vi "getAdditionalDataFromXML.vi"(8 "error in (no error)":errorcluster, 10 "Xml":refnum<class "xmlNode.lvclass">, 11 "SingleToneRamp in":refnum<class "SingleToneRamp.lvclass">) -> (0 "error out":errorcluster, 2 "Xml out":refnum<class "xmlNode.lvclass">, 3 "SingleToneRamp out":refnum<class "SingleToneRamp.lvclass">)   [LabVIEW 2009, in "Tools.lvlib" / "Scripting.lvlib" / "SingleToneRamp.lvclass"]
uses:
  SingleToneRamp.lvclass
  xmlNode/xmlNode.lvclass
  SingleToneRamp.lvclass/SingleToneRamp.ctl
  SingleTone.lvclass
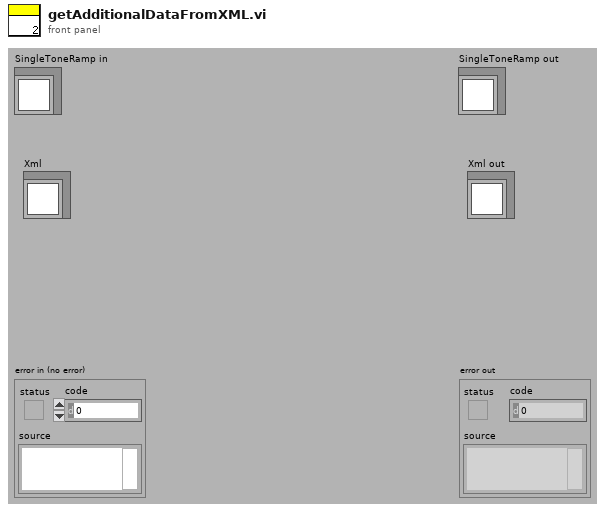
[diagram p1: front panel]
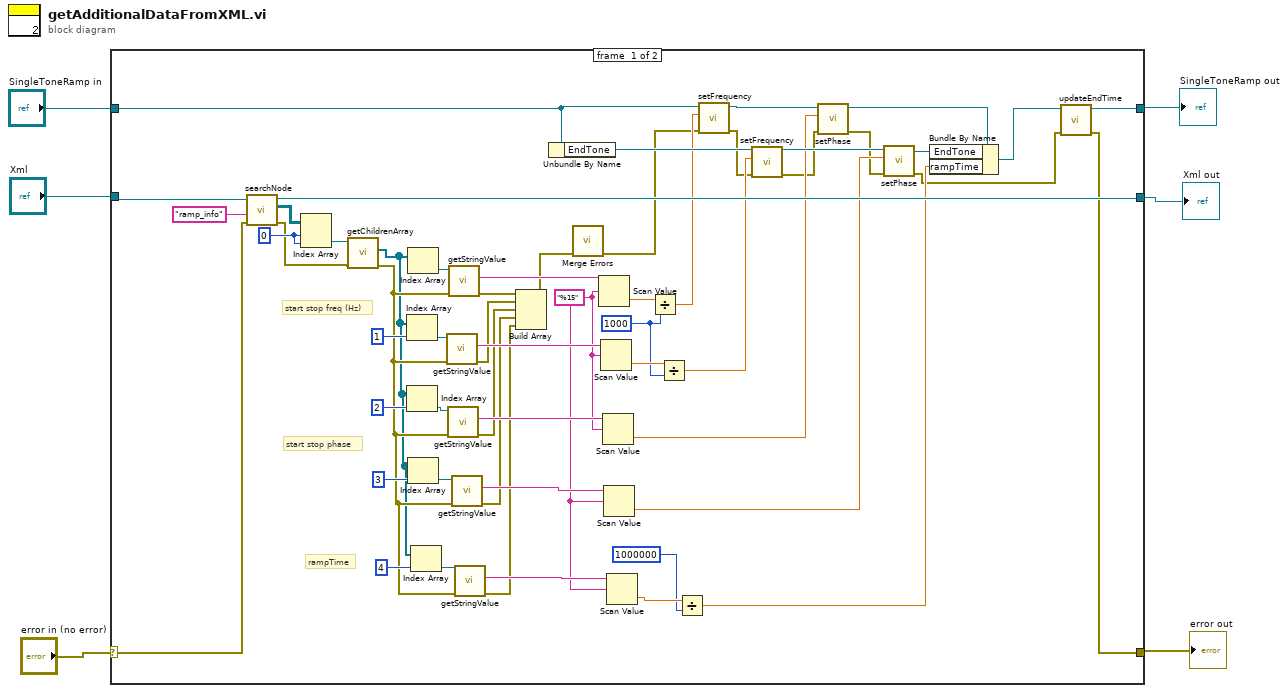
[diagram p0: block diagram]
diagram:
  n1 = case shown="No Error" "error in (no error)" {
    selector: "error in (no error)" -> [w15 w63]
    tunnel: [w14 w63] -> w5
    tunnel: [w17 w62] -> w3
    tunnel: "SingleToneRamp in" -> [w32 w62]
    tunnel: "Xml" -> [w47 _]
    tunnel: [w46 _] -> w1
    frame #0 {
      w44 = 1000
      w35 = "%15"
      w59 = 0
      # "rampTime"
      # "start stop freq (Hz)"
      # "start stop phase"
      n2 = call-dynamic "searchNode.vi"("error in (no error)"=w15, "searchElementName"="ramp_info", "xmlNode in"=w47) -> ("error out"=w57:errorcluster, "arrayXmlNodes"=w60:refnum<class "xmlNode.lvclass">[][], "xmlNode out"=w46:refnum<class "xmlNode.lvclass">)  [unwired: 6 in]
      n3 = Index Array(array=w60, index (row)=w59, index (col)=w59) -> (element=w58:refnum<class "xmlNode.lvclass">)
      n4 = call-dynamic "getChildrenArray.vi"("error in (no error)"=w57, "xmlNode.lvclass in"=w58) -> ("error out"=w37:errorcluster, "Children"=w36:refnum<class "xmlNode.lvclass">[])  [unwired: 7 in, 1 out]
      n5 = Index Array(array=w36, index=1) -> (element=w55:refnum<class "xmlNode.lvclass">)
      n6 = Index Array(array=w36, index=2) -> (element=w53:refnum<class "xmlNode.lvclass">)
      n7 = Index Array(array=w36) -> (element=w56:refnum<class "xmlNode.lvclass">)  [unwired: 1 in]
      n8 = Index Array(array=w36, index=3) -> (element=w41:refnum<class "xmlNode.lvclass">)
      n9 = Index Array(array=w36, index=4) -> (element=w38:refnum<class "xmlNode.lvclass">)
      n10 = call-dynamic "getStringValue.vi"("error in (no error)"=w37, "xmlNode.lvclass in"=w55) -> ("error out"=w12:errorcluster, "stringValue"=w50:string)  [unwired: 7 in, 1 out]
      n11 = call-dynamic "getStringValue.vi"("error in (no error)"=w37, "xmlNode.lvclass in"=w53) -> ("error out"=w11:errorcluster, "stringValue"=w48:string)  [unwired: 7 in, 1 out]
      n12 = call-dynamic "getStringValue.vi"("error in (no error)"=w37, "xmlNode.lvclass in"=w56) -> ("error out"=w13:errorcluster, "stringValue"=w51:string)  [unwired: 7 in, 1 out]
      n13 = call-dynamic "getStringValue.vi"("error in (no error)"=w37, "xmlNode.lvclass in"=w41) -> ("error out"=w10:errorcluster, "stringValue"=w42:string)  [unwired: 7 in, 1 out]
      n14 = call-dynamic "getStringValue.vi"("error in (no error)"=w37, "xmlNode.lvclass in"=w38) -> ("error out"=w9:errorcluster, "stringValue"=w39:string)  [unwired: 7 in, 1 out]
      n15 = Build Array(w13, w12, w11, w10, w9) -> (w8:errorcluster[])
      n16 = Unbundle By Name(w32) -> ("EndTone"=w31:refnum<class "SingleTone.lvclass">)
      n17 = call <vilib>:"Merge Errors.vi"("error array in"=w8) -> ("error out"=w7:errorcluster)  [unwired: 6 in]
      n18 = Scan Value(string=w51, format string=w35) -> (value=w49:dbl)  [unwired: 1 in, 1 out]
      n19 = Scan Value(string=w50, format string=w35) -> (value=w45:dbl)  [unwired: 1 in, 1 out]
      n20 = Scan Value(string=w48, format string=w35) -> (value=w25:dbl)  [unwired: 1 in, 1 out]
      n21 = Scan Value(string=w42, format string=w35) -> (value=w24:dbl)  [unwired: 1 in, 1 out]
      n22 = Scan Value(string=w39, format string=w35) -> (value=w34:dbl)  [unwired: 1 in, 1 out]
      n23 = Divide(x=w49, y=w44) -> (x/y=w30:dbl)
      n24 = Divide(x=w45, y=w44) -> (x/y=w29:dbl)
      n25 = Divide(x=w34, y=1000000) -> (x/y=w19:dbl)
      n26 = call "setFrequency.vi"("error in (no error)"=w7, "frequency"=w30, "SingleTone.lvclass in"=w32) -> ("error out"=w28:errorcluster, "SingleTone.lvclass out"=w27:refnum<class "SingleToneRamp.lvclass">)  [unwired: 7 in]
      n27 = call "setFrequency.vi"("error in (no error)"=w28, "frequency"=w29, "SingleTone.lvclass in"=w31) -> ("error out"=w23:errorcluster, "SingleTone.lvclass out"=w26:refnum<class "SingleTone.lvclass">)  [unwired: 7 in]
      n28 = call "setPhase.vi"("error in (no error)"=w23, "phase"=w25, "SingleTone.lvclass in"=w27) -> ("error out"=w22:errorcluster, "SingleTone.lvclass out"=w21:refnum<class "SingleToneRamp.lvclass">)  [unwired: 7 in]
      n29 = call "setPhase.vi"("error in (no error)"=w22, "phase"=w24, "SingleTone.lvclass in"=w26) -> ("error out"=w16:errorcluster, "SingleTone.lvclass out"=w20:refnum<class "SingleTone.lvclass">)  [unwired: 7 in]
      n30 = Bundle By Name(cluster=w21, "EndTone"=w20, "rampTime"=w19) -> (w18:refnum<class "SingleToneRamp.lvclass">)
      n31 = call-dynamic "updateEndTime.vi"("error in (no error)"=w16, "SingleToneRamp in"=w18) -> ("error out"=w14:errorcluster, "SingleToneRamp out"=w17:refnum<class "SingleToneRamp.lvclass">)  [unwired: 8 in]
    }
    frame #1 {
    }
  }
  "error out" <- w5
  "SingleToneRamp out" <- w3
  "Xml out" <- w1
